vi "Update Library Version.vi"(6 "Changes":string, 8 "error in (no error)":errorcluster, 9 "Version":T1, 10 "Search Pattern":string, 11 "LabVIEW Build Script in":refnum<class "LabVIEW Build Script.lvclass">) -> (0 "error out":errorcluster, 1 "Description":string, 3 "LabVIEW Build Script out":refnum<class "LabVIEW Build Script.lvclass">)   [LabVIEW 2021, in "LabVIEW Build Script.lvclass"]
uses:
  LabVIEW Build Script.lvclass
  LabVIEW Build Script.lvclass/LabVIEW Build Script.ctl
  <vilib>/CIF Foundation/CIF Utilities/Errors/Errors_CIF_U.lvlib
  Build Script Common/Typedef/Build Script Errors.ctl
  Build Script Common/Build Script Common.lvlib
  <vilib>/CIF Foundation/CIF LabVIEW Scripting/LV Scripting/LV Scripting Utilities.lvlib
  <vilib>/CIF Foundation/CIF LabVIEW Scripting/LV Scripting/Typedef/Version.ctl
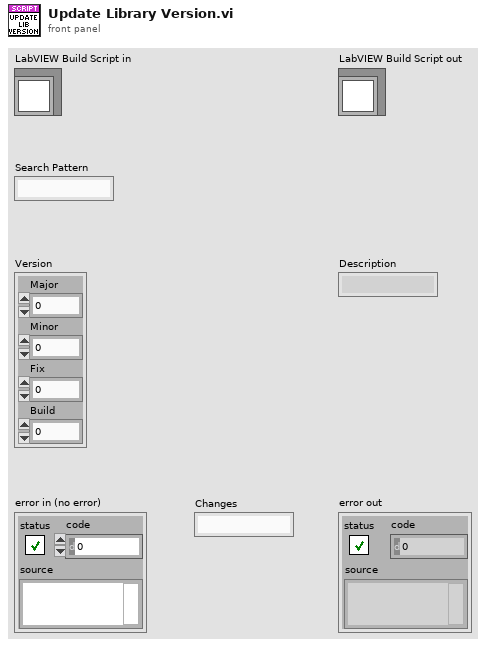
[diagram p1: front panel]
types:
  T1 = typedef "Version.ctl" = cluster{"Major":u16, "Minor":u16, "Fix":u16, "Build":u16}
  T2 = typedef "Build Script Common.lvlib/Build Script Errors.ctl" = enum16{"Item not found"}
  T3 = typedef "LV Scripting Utilities.lvlib/Library Map.ctl" = map{string, refnum<vi>}
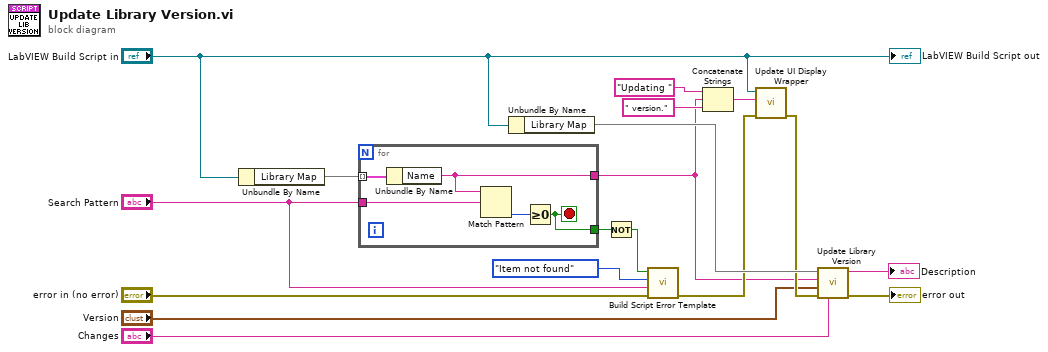
[diagram p0: block diagram]
diagram:
  n1 = Unbundle By Name("LabVIEW Build Script in") -> ("Library Map"=w15:T3)
  n2 = for {
    tunnel: w15 -> [w23] mode=indexing
    tunnel: "Search Pattern" -> [w22]
    tunnel: [w20] -> w4
    tunnel: [w19] -> w13
    stop <- w19 stop-if-true
    n3 = Unbundle By Name(w23) -> ("Name"=w20:string)
    n4 = Match Pattern(string=w20, regular expression=w22) -> (offset past match=w21:i32)  [unwired: 1 in, 3 out]
    n5 = Greater Or Equal To 0?(x=w21) -> (x >= 0?=w19:bool)
  }
  n6 = Unbundle By Name("LabVIEW Build Script in") -> ("Library Map"=w9:T3)
  n7 = Not(x=w13) -> (.not. x?=w12:bool)
  n8 = call "Build Script Error Template.vi"("error in (no error)"="error in (no error)", "String to Append"="Search Pattern", "Error"=Build_Script_Errors."Item not found", "Insert Error"=w12) -> ("error out"=w7:errorcluster)  [unwired: 7 in]
  n9 = Concatenate Strings("Updating " ("Update for Display"), w4, " version." ("string")) -> (w17:string)
  n10 = call "Update UI Display Wrapper.vi"("error in (no error)"=w7, "Update for Display"=w17, "LabVIEW Build Script in"="LabVIEW Build Script in") -> ("error out"=w6:errorcluster)  [unwired: 8 in]
  n11 = call <vilib>:"Update Library Version.vi"("Changes"="Changes", "error in (no error)"=w6, "New Version"="Version", "Library Name"=w4, "Library Map"=w9) -> ("error out"=→"error out":errorcluster, "Description"=→"Description":string)  [unwired: 5 in]
  "LabVIEW Build Script out" <- "LabVIEW Build Script in"
